vi "Parse Value.vi"(8 "error in (no error)":errorcluster, 11 "String":string) -> (0 "error out":errorcluster, 3 "Value":variant)   [LabVIEW 2015, in "YAML Parser.lvclass"]
uses:
  YAML Parser.lvclass
  YAML Type.ctl
panel:
  out "empty?":bool
  out "YAML Type":T1
  out "value":dbl
  out "output string":string
  out "Value 2":string
  out "Key 2":string
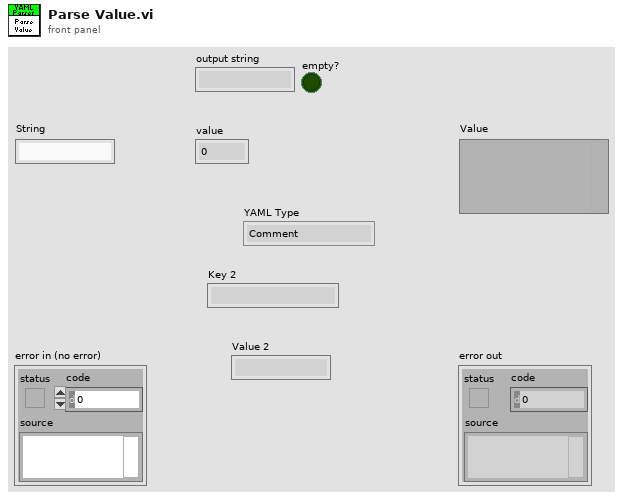
[diagram p1: front panel]
types:
  T1 = typedef "YAML Parser.lvclass/YAML Type.ctl" = enum16{"Comment", "Null", "Integer", "Float", "String", "Multilines String", "Boolean", "Object", "Array", "Reference"}
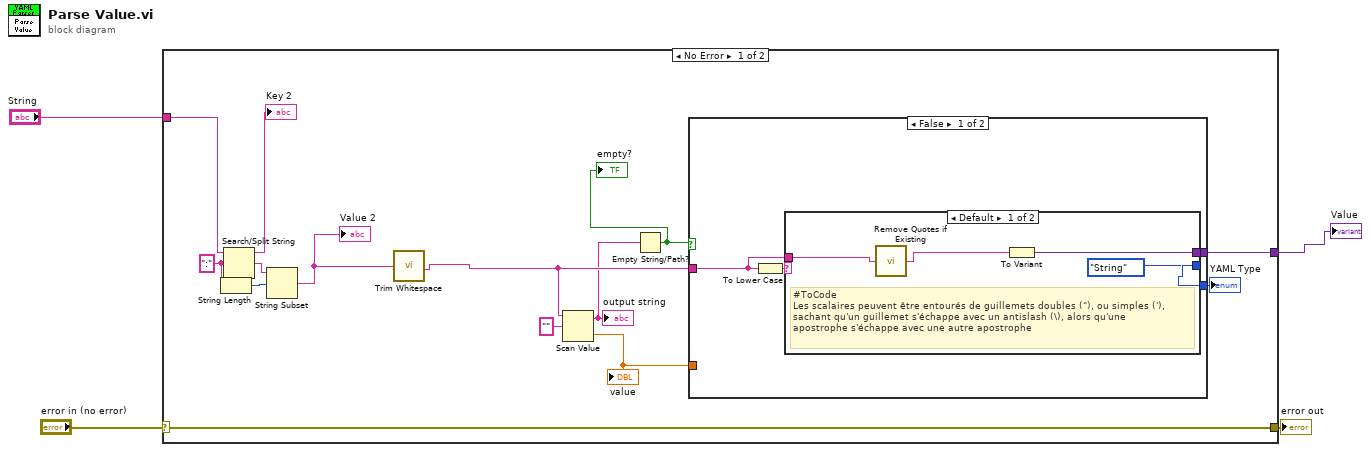
[diagram p0: block diagram]
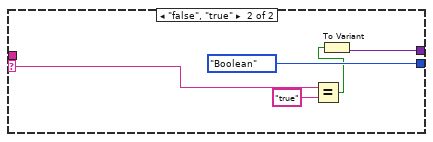
[diagram p2: hidden frame]
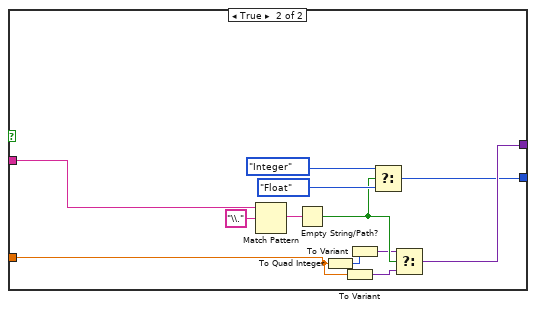
[diagram p3: hidden frame]
diagram:
  n1 = case shown="No Error" "error in (no error)" {
    selector: "error in (no error)" -> [w18 w44]
    tunnel: [w18 w44] -> w3
    tunnel: "String" -> [w16 _]
    tunnel: [w15 _] -> w1
    frame No Error {
      w7 = ":" ("search string/char (-)")
      n2 = String Length(string=w7) -> (length=w6:i32)
      n3 = Search/Split String(string=w16, search string/char (-)=w7) -> (substring before match=→"Key 2":string, match + rest of string=w8:string)  [unwired: 1 in, 1 out]
      n4 = String Subset(string=w8, offset (0)=w6) -> (substring=w5:string)  [unwired: 1 in]
      "Value 2" <- w5
      n5 = call <vilib>:"Trim Whitespace.vi"("string"=w5) -> ("trimmed string"=w14:string)  [unwired: 1 in]
      n6 = Scan Value(string=w14, format string="") -> (output string=w13:string, value=w11:dbl)  [unwired: 1 in]
      "output string" <- w13
      "value" <- w11
      n7 = Empty String/Path?(string/path=w13) -> (empty?=w12:bool)
      "empty?" <- w12
      n8 = case shown="False" w12 {
        tunnel: [w21 w35] -> w15
        tunnel: w14 -> [w20 w39]
        tunnel: w11 -> [_ w36]
        tunnel: [w19 w34] -> w9
        frame False {
          n9 = To Lower Case(string=w20) -> (all lower case string=w22:string)
          n10 = case shown="Default" w22 {
            selector: w22 -> [_ w29]
            tunnel: [YAML_Type."String" ("YAML Type") YAML_Type."Boolean" ("YAML Type")] -> w19
            tunnel: [w25 w30] -> w21
            tunnel: w20 -> [w24 _]
            frame Default {
              # "#ToCode\nLes scalaires peuvent être entourés de guillemets doubles (\"), ou simples ('), \nsachant qu'un guillemet s'échappe avec un antislash (\\), alors qu'une \napostrophe s'échappe avec une autre apostrophe"
              n11 = call "Remove Quotes if Existing.vi"("String"=w24) -> ("String out"=w23:string)
              n12 = To Variant(anything=w23) -> (Variant=w25:variant)
            }
            frame "false", "true" {
              n13 = Equal?(x=w29, y="true") -> (x = y?=w27:bool)
              n14 = To Variant(anything=w27) -> (Variant=w30:variant)
            }
          }
        }
        frame True {
          n15 = Match Pattern(string=w39, regular expression="\\.") -> (match substring=w42:string)  [unwired: 1 in, 3 out]
          n16 = Empty String/Path?(string/path=w42) -> (empty?=w37:bool)
          n17 = To Quad Integer(1:w36) -> (0:w38:i64)
          n18 = To Variant(anything=w36) -> (Variant=w32:variant)
          n19 = To Variant(anything=w38) -> (Variant=w33:variant)
          n20 = Select(t=YAML_Type."Integer" ("YAML Type"), s=w37, f=YAML_Type."Float" ("YAML Type")) -> (s? t:f=w34:T1)
          n21 = Select(t=w33, s=w37, f=w32) -> (s? t:f=w35:variant)
        }
      }
      "YAML Type" <- w9
    }
    frame Error {
    }
  }
  "error out" <- w3
  "Value" <- w1
